vi "Control many leds By switches.vi"() -> ()   [LabVIEW 2019]
uses:
  <vilib>/LabVIEW Interface for Arduino/Type Defs/Board Type.ctl
  <vilib>/LabVIEW Interface for Arduino/Type Defs/Connection Type.ctl
  <vilib>/LabVIEW Interface for Arduino/Type Defs/Pin Mode.ctl
  <vilib>/LabVIEW Interface for Arduino/LabVIEW Interface for Arduino.lvlib
panel:
  in  "stop":bool
  in  "VISA resource":refnum<visa-resource-name>
  in  "Boolean 3":bool
  in  "Boolean 2":bool
  in  "Boolean":bool
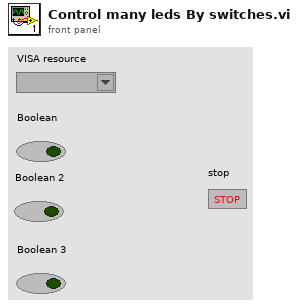
[diagram p1: front panel]
types:
  T1 = typedef "LabVIEW Interface for Arduino.lvlib/Pin Mode.ctl" = enum8{"Input", "Output"}
  T2 = typedef "LabVIEW Interface for Arduino.lvlib/Connection Type.ctl" = enum8{"USB / Serial", "XBEE", "BlueSmirf (Bluetooth)"}
  T3 = typedef "LabVIEW Interface for Arduino.lvlib/Board Type.ctl" = enum16{"Uno", "Dimuelanove w/Atmega 328", "Mega 2560"}
  T4 = typedef "LabVIEW Interface for Arduino.lvlib/Arduino Resource.ctl" = cluster{"VISA resource":refnum<visa-resource-name>, "Board Type":T3, "Connection Type":enum8{"USB / Serial"}, "Bytes Per Packet (15)":u8}
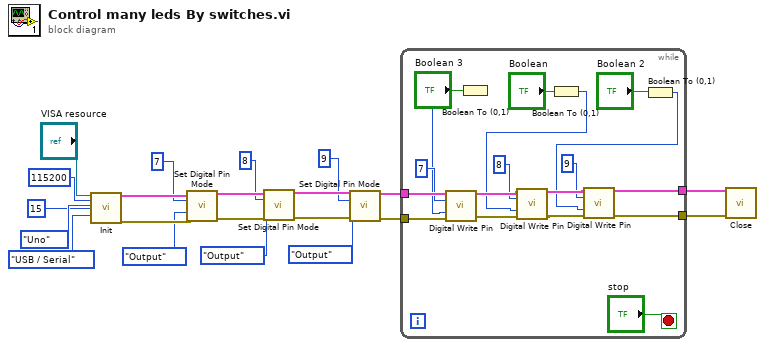
[diagram p0: block diagram]
diagram:
  n1 = call <vilib>:"Init.vi"("VISA resource"="VISA resource", "Baud Rate (115200)"=u32 115200, "Board Type (Uno)"=Board_Type."Uno", "Bytes Per Packet (15)"=u32 15, "Connection Type (USB/Serial)"=Connection_Type."USB / Serial") -> ("Arduino Resource"=w16:T4, "error out"=w13:errorcluster)  [unwired: 13 in]
  n2 = call <vilib>:"Set Digital Pin Mode.vi"("Arduino Resource"=w16, "Digital I/O Pin"=u8 7, "Pin Mode (Input)"=Pin_Mode."Output", "error in"=w13) -> ("Arduino Resource"=w15:T4, "error out"=w12:errorcluster)  [unwired: 10 in]
  n3 = call <vilib>:"Set Digital Pin Mode.vi"("Arduino Resource"=w15, "Digital I/O Pin"=u8 8, "Pin Mode (Input)"=Pin_Mode."Output", "error in"=w12) -> ("Arduino Resource"=w14:T4, "error out"=w11:errorcluster)  [unwired: 10 in]
  n4 = call <vilib>:"Set Digital Pin Mode.vi"("Arduino Resource"=w14, "Digital I/O Pin"=u8 9, "Pin Mode (Input)"=Pin_Mode."Output", "error in"=w11) -> ("Arduino Resource"=w10:T4, "error out"=w9:errorcluster)  [unwired: 10 in]
  n5 = while {
    tunnel: w10 -> [w38]
    tunnel: w9 -> [w33]
    tunnel: [w32] -> w8
    tunnel: [w31] -> w7
    stop <- "stop" stop-if-true
    n6 = Boolean To (0,1)(Boolean="Boolean 3") -> (0, 1=w24:i16)
    n7 = call <vilib>:"Digital Write Pin.vi"("Arduino Resource"=w38, "Digital I/O Pin (0)"=u8 7, "Value (0)"=w24, "error in"=w33) -> ("Arduino Resource"=w37:T4, "error out"=w34:errorcluster)  [unwired: 10 in]
    n8 = Boolean To (0,1)(Boolean="Boolean") -> (0, 1=w23:i16)
    n9 = call <vilib>:"Digital Write Pin.vi"("Arduino Resource"=w37, "Digital I/O Pin (0)"=u8 8, "Value (0)"=w23, "error in"=w34) -> ("Arduino Resource"=w36:T4, "error out"=w35:errorcluster)  [unwired: 10 in]
    n10 = Boolean To (0,1)(Boolean="Boolean 2") -> (0, 1=w22:i16)
    n11 = call <vilib>:"Digital Write Pin.vi"("Arduino Resource"=w36, "Digital I/O Pin (0)"=u8 9, "Value (0)"=w22, "error in"=w35) -> ("Arduino Resource"=w32:T4, "error out"=w31:errorcluster)  [unwired: 10 in]
  }
  n12 = call <vilib>:"Close.vi"("Arduino Resource"=w8, "error in"=w7) -> ()  [unwired: 13 in, 1 out]
